vi "Generate Apriltag Image Data (TagCustom48h12).vi"(7 "Add Border (Default: False)":bool, 8 "error in (no error)":errorcluster, 11 "ID":i32) -> (0 "error out":errorcluster, 1 "Alpha":u8[][](array[numeric]), 3 "Tag Image Data":u8[][](array[numeric]) format="%.0x")   [LabVIEW 2020, in "feature_detection.lvlib"]
doc: "Generate the AprilTag Image Data for a specified Tag ID. Use Apriltag Tag ID List.vi to get a list of valid Tag IDs for each Tag Family."
uses:
  feature_detection.lvlib
  TagIDOutOfRangeError.vi
  TagSetPixel.vi
  TagRotatePixelArray.vi
  <vilib>/Utility/error.llb/Error Cluster From Error Code.vi
  TagLayoutConvert.vi
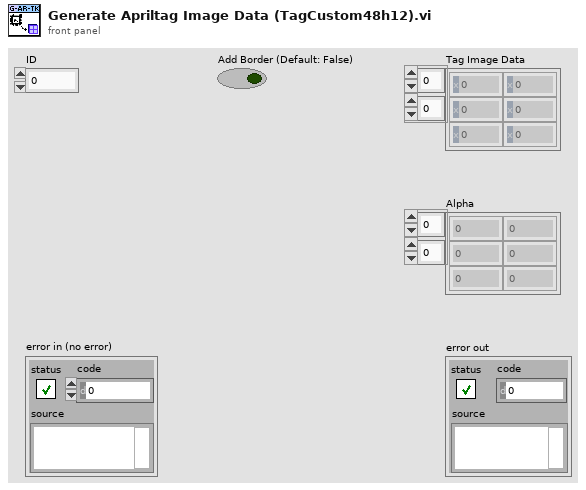
[diagram p1: front panel]
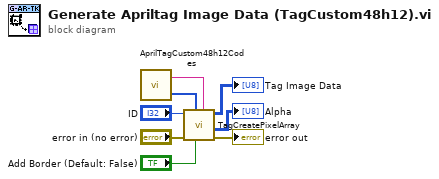
[diagram p0: block diagram]
diagram:
  n1 = call "AprilTagCustom48h12Codes.vi"() -> ("Codes"=w3:i64[], "Layout"=w4:string)  [unwired: 2 in]
  n2 = call "TagCreatePixelArray.vi"("Layout"=w4, "Add Border"="Add Border (Default: False)", "Codes"=w3, "error in (no error)"="error in (no error)", "ID"="ID") -> ("error out"=→"error out":errorcluster, "Alpha"=→"Alpha":u8[][], "Pixels"=→"Tag Image Data":u8[][])  [unwired: 4 in]
